vi "CanOpen Schließen.vi"(8 "error in (no error)":errorcluster, 10 "CanOpen Obj":T1={"node-ID"=1, "RPDO1 object"=refnum, "TPDO1 object"=refnum, "RPDO2 object"=refnum, "TPDO2 object"=refnum, "SYNC object"=refnum}) -> (0 "Fehler (Ausgang)":errorcluster)   [LabVIEW 2014]
uses:
  <vilib>/CANopenLib/CANOPEN.llb/CANopen TPDO Close.vi
  <vilib>/CANopenLib/CANOPEN.llb/CANopen RPDO Close.vi
  <vilib>/CANopenLib/CANOPEN.llb/CANopen SYNC Close.vi
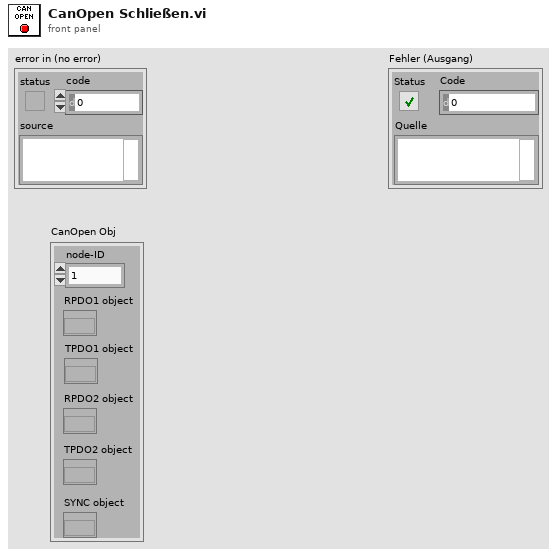
[diagram p1: front panel]
types:
  T1 = cluster{"node-ID":u8, "RPDO1 object":refnum<k20>, "TPDO1 object":refnum<k20>, "RPDO2 object":refnum<k20>, "TPDO2 object":refnum<k20>, "SYNC object":refnum<k20>}
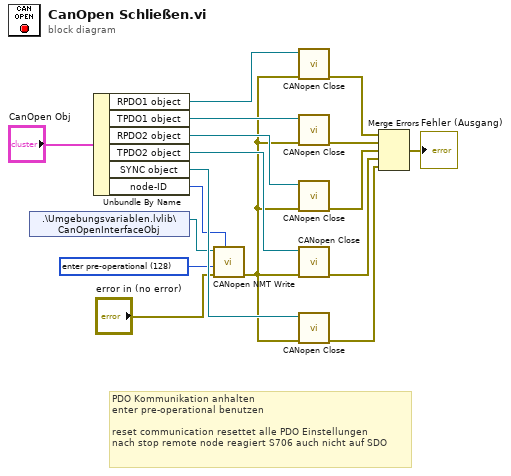
[diagram p0: block diagram]
diagram:
  w4 = u16 128 items=["start remote node"=1, "stop remote node"=2, "enter pre-operational"=128, "reset node"=129, "reset communication"=130] ("command")
  # "PDO Kommunikation anhalten\nenter pre-operational benutzen\n\nreset communication resettet alle PDO Einstellungen\nnach stop remote node reagiert S706 auch nicht auf SDO"
  n1 = shared-variable ".\\Umgebungsvariablen.lvlib\\CanOpenInterfaceObj"() -> (w8:refnum<k20>)  [unwired: 1 in, 1 out]
  n2 = Unbundle By Name("CanOpen Obj") -> ("RPDO1 object"=w7:refnum<k20>, "TPDO1 object"=w6:refnum<k20>, "RPDO2 object"=w16:refnum<k20>, "TPDO2 object"=w15:refnum<k20>, "SYNC object"=w14:refnum<k20>, "node-ID"=w5:u8)
  n3 = call <vilib>:"CANopen NMT Write.vi"("node-ID (0)"=w5, "error in (no error)"="error in (no error)", "command"=w4, "interface object in"=w8) -> ("error out"=w3:errorcluster)  [unwired: 6 in, 1 out]
  n4 = call-poly <vilib>:"CANopen Close.vi"("error in (no error)"=w3, "RPDO object in"=w7) -> ("error out"=w2:errorcluster)  [unwired: 9 in]
  n5 = call-poly <vilib>:"CANopen Close.vi"("error in (no error)"=w3, "TPDO object in"=w6) -> ("error out"=w1:errorcluster)  [unwired: 9 in]
  n6 = call-poly <vilib>:"CANopen Close.vi"("error in (no error)"=w3, "RPDO object in"=w16) -> ("error out"=w13:errorcluster)  [unwired: 9 in]
  n7 = call-poly <vilib>:"CANopen Close.vi"("error in (no error)"=w3, "TPDO object in"=w15) -> ("error out"=w12:errorcluster)  [unwired: 9 in]
  n8 = call-poly <vilib>:"CANopen Close.vi"("error in (no error)"=w3, "SYNC object in"=w14) -> ("error out"=w11:errorcluster)  [unwired: 9 in]
  n9 = Merge Errors(w2, w1, w13, w12, w11) -> (→"Fehler (Ausgang)":errorcluster)
